vi "DSF.Transceiver.UDP.Rx.Update Transfer.vi"(8 "error in (no error)":errorcluster, 9 "data":string, 10 "Transfer":refnum<class "DSF.Engine.Transfer.lvclass">, 11 "UDP Transceiver in":refnum<class "DSF.Transceiver.UDP.lvclass">) -> (0 "error out":errorcluster, 3 "UDP Transceiver out":refnum<class "DSF.Transceiver.UDP.lvclass">)   [LabVIEW 2017, in "DSF.Transceiver.UDP.lvlib" / "DSF.Transceiver.UDP.lvclass"]
uses:
  DSF.Transceiver.UDP.lvclass
  Built/Engine/DSF.Engine.lvlibp/Engine/Classes/Transfer/DSF.Engine.Transfer.lvclass
  DSF.Transceiver.UDP.Errors.Rx.Size Mismatch.vi
  <vilib>/NI/Static Error Handling/VIs/Static Error Handling.Source Buffer.Write.String.vi
  <vilib>/NI/Static Error Handling/VIs/Static Error Handling.Source Buffer.Write.Numeric.Scalar.Base10.vi
  <vilib>/NI/Static Error Handling/VIs/Static Error Handling.Source Buffer.Write.Numeric.Scalar.Base10 (U64).vi
  Built/Engine/DSF.Engine.lvlibp/Engine/Classes/Buffer/DSF.Engine.Memory.Buffer.Write.1D.U8.vi
  DSF.Transceiver.UDP.Error.Create.vi
  Built/Engine/DSF.Engine.lvlibp/Engine/Classes/Buffer/DSF.Engine.Memory.Buffer.lvclass
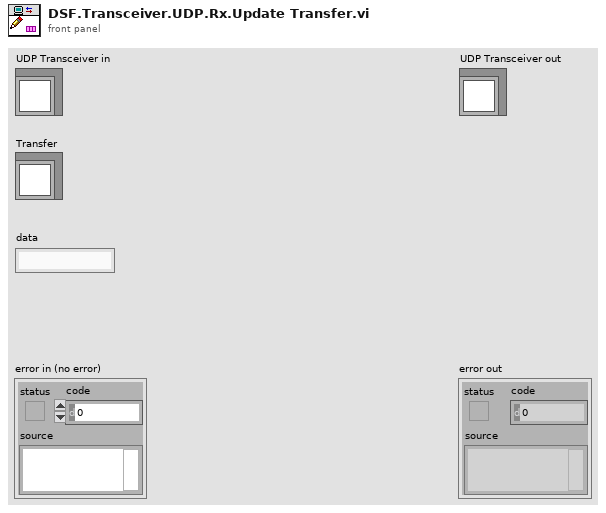
[diagram p1: front panel]
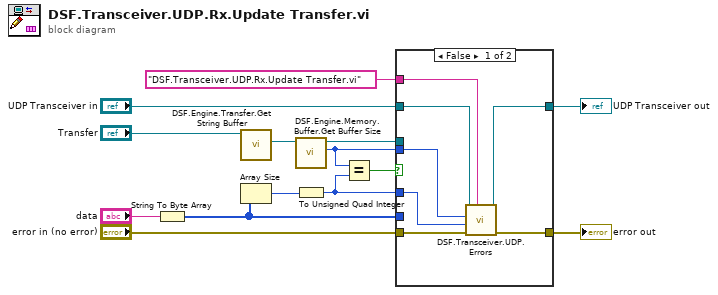
[diagram p0: block diagram]
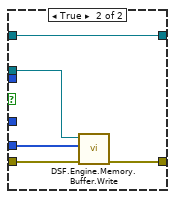
[diagram p2: hidden frame]
diagram:
  n1 = String To Byte Array(string="data") -> (unsigned byte array=w7:u8[])
  n2 = call "DSF.Engine.Transfer.Get String Buffer.vi"("Transfer in"="Transfer") -> ("Buffer"=w14:refnum<class "DSF.Engine.Memory.Buffer.lvclass">)  [unwired: 9 in, 1 out]
  n3 = Array Size(array=w7) -> (size(s)=w13:i32)
  n4 = call "DSF.Engine.Memory.Buffer.Get Buffer Size.vi"("Buffer in"=w14) -> ("buffer size"=w3:u64, "Buffer out"=w12:refnum<class "DSF.Engine.Memory.Buffer.lvclass">)  [unwired: 9 in]
  n5 = To Unsigned Quad Integer(1:w13) -> (0:w2:u64)
  n6 = Equal?(x=w3, y=w2) -> (x = y?=w4:bool)
  n7 = case shown="False" w4 {
    tunnel: w12 -> [_ w26]
    tunnel: "error in (no error)" -> [w21 w25]
    tunnel: [w20 w24] -> w9
    tunnel: w7 -> [_ w23]
    tunnel: "UDP Transceiver in" -> [w19 w22]
    tunnel: [w18 w22] -> w5
    tunnel: w3 -> [w16 _]
    tunnel: w2 -> [w17 _]
    tunnel: "DSF.Transceiver.UDP.Rx.Update Transfer.vi" ("source vi name") -> [w15 _]
    frame False {
      n8 = call-poly "DSF.Transceiver.UDP.Errors.vi"("source vi name"=w15, "error in (no error)"=w21, "actual size"=w17, "expected size"=w16, "UDP Transceiver in"=w19) -> ("error out"=w20:errorcluster, "UDP Transceiver out"=w18:refnum<class "DSF.Transceiver.UDP.lvclass">)  [unwired: 5 in]
    }
    frame True {
      n9 = call-poly "DSF.Engine.Memory.Buffer.Write.vi"("error in (no error)"=w25, "buffer in"=w23, "Buffer in"=w26) -> ("error out"=w24:errorcluster)  [unwired: 5 in, 3 out]
    }
  }
  "error out" <- w9
  "UDP Transceiver out" <- w5
